vi "HeaderAction.vi"(0 "InstrClass":refnum<class "Spex.lvclass"> caption="DNL_LabVIEW Object in", 11 "error in (no error)":errorcluster caption="entrée d'erreur (pas d'erreur)") -> (4 "InstrClassOut":refnum<class "Spex.lvclass"> caption="DNL_LabVIEW Object out", 6 "DataNames":string[](array[string]), 8 "Instr Name":string, 10 "HeaderString":string, 14 "DisplayNames":string[](array[string]), 15 "error out":errorcluster caption="sortie d'erreur")   [LabVIEW 2019, in "Spex.lvclass"]
uses:
  Spex.lvclass
  C:/Programmes Labview/LabScanV1A/DevicesClass/BaseDevice/BaseDevice.lvclass
  Spex.lvclass/Spex.ctl
  BaseDevice/BaseDevice.lvclass
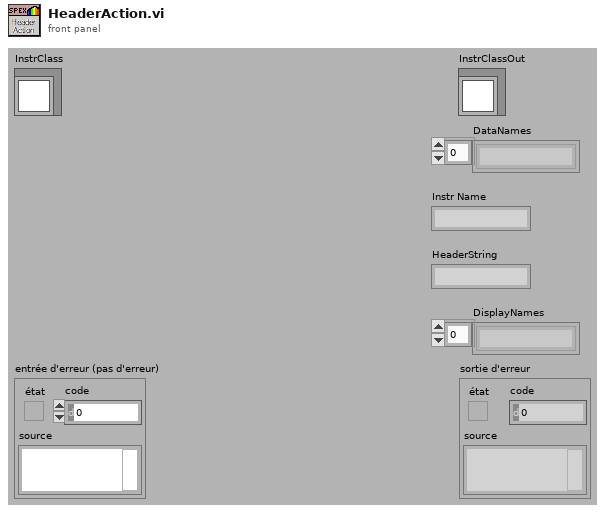
[diagram p1: front panel]
types:
  T1 = typedef "Spex.lvclass/Spex_Func.ctl" = enum16{"Position (nm)"}
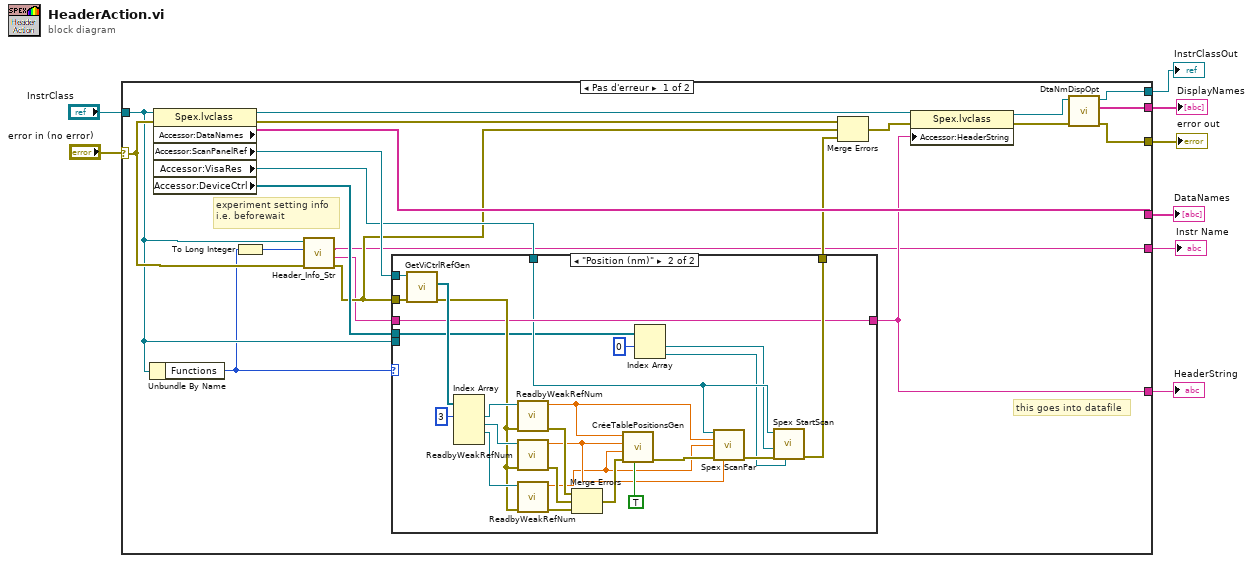
[diagram p0: block diagram]
diagram:
  n1 = case shown="Pas d'erreur" "error in (no error)" {
    selector: "error in (no error)" -> [w15 w57]
    tunnel: [w26 _] -> w7
    tunnel: [w29 _] -> w6
    tunnel: "InstrClass" -> [w14 w58]
    tunnel: [w24 w57] -> w4
    tunnel: [w23 w58] -> w2
    tunnel: [w10 _] -> w3
    tunnel: [w21 _] -> w1
    frame No Error {
      # "this goes into datafile"
      # "experiment setting info\ni.e. beforewait"
      n2 = Unbundle By Name(w14) -> ("Functions"=w13:T1)
      n3 = property class="Spex.lvclass"(reference=w14, error in=w15) -> (reference out=w28:refnum<class "Spex.lvclass">, error out=w27:errorcluster, "Accessor:DataNames"=w29:string[], "Accessor:ScanPanelRef"=w19:refnum<vi>, "Accessor:VisaRes"=w17:refnum<visa-resource-name>, "Accessor:DeviceCtrl"=w16:refnum<vi>[])
      n4 = To Long Integer(number=w13) -> (32bit integer=w12:i32)
      n5 = call-dynamic "Header_Info_Str.vi"("error in (no error)"=w15, "Functions"=w12, "DefaultDev in"=w14) -> ("error out"=w11:errorcluster, "HdrInfoStr"=w9:string, "InstrumentName"=w10:string)  [unwired: 5 in, 1 out]
      n6 = case shown="\"Position (nm)\"" w13 {
        tunnel: [w31 w38] -> w26
        tunnel: w9 -> [w31 w38]
        tunnel: w14 -> [_ _]
        tunnel: w19 -> [_ w52]
        tunnel: w11 -> [w30 w51]
        tunnel: [w30 w39] -> w18
        tunnel: w17 -> [_ w37]
        tunnel: w16 -> [_ w35]
        frame Default {
        }
        frame "Position (nm)" {
          n7 = call <userlib>:"GetViCtrlRefGen.vi"("ErrorIn(No Error)"=w51, "VIRef"=w52) -> ("sortie d'erreur"=w49:errorcluster, "ControlsRefs"=w50:refnum<vi>[])  [unwired: 7 in, 1 out]
          n8 = Index Array(array=w50, index #1=3 ("indice")) -> (element #1=w56:refnum<vi>, element #2=w55:refnum<vi>, element #3=w53:refnum<vi>)  [unwired: 3 in, 1 out]
          n9 = call <userlib>:"ReadbyWeakRefNum.vi"("error in"=w49, "Control Ref"=w56) -> ("error out"=w47:errorcluster, "Valeur"=w42:dbl)  [unwired: 8 in]
          n10 = call <userlib>:"ReadbyWeakRefNum.vi"("error in"=w49, "Control Ref"=w55) -> ("error out"=w45:errorcluster, "Valeur"=w41:dbl)  [unwired: 8 in]
          n11 = call <userlib>:"ReadbyWeakRefNum.vi"("error in"=w49, "Control Ref"=w53) -> ("error out"=w44:errorcluster, "Valeur"=w36:dbl)  [unwired: 8 in]
          n12 = Merge Errors(w47, w45, w44) -> (w46:errorcluster)
          n13 = call "CréeTablePositionsGen.vi"("InvInt"=TRUE, "error in (no error)"=w46, "Fin"=w36, "Increment"=w41, "Debut"=w42) -> ("error out"=w43:errorcluster)  [unwired: 4 in, 2 out]
          n14 = Index Array(array=w35, index #1=0 ("indice")) -> (element #1=w33:refnum<vi>, element #2=w32:refnum<vi>)  [unwired: 1 in]
          n15 = call <userlib>:"Spex ScanPar.vi"("Port"=w37, "Start(nm)"=w42, "End(nm)"=w36, "error in"=w43, "Step (nm)"=w41) -> ("error out"=w40:errorcluster)  [unwired: 10 in]
          n16 = call <userlib>:"Spex StartScan.vi"("Moving Ref"=w32, "error in"=w40, "Lambda Ref"=w33, "Port"=w37) -> ("error out"=w39:errorcluster)  [unwired: 5 in, 2 out]
        }
      }
      n17 = Merge Errors(w27, w11, w18) -> (w20:errorcluster)
      n18 = property class="Spex.lvclass"(reference=w28, error in=w20, "Accessor:HeaderString"=w26) -> (reference out=w22:refnum<class "Spex.lvclass">, error out=w25:errorcluster)
      n19 = call "DtaNmDispOpt.vi"("error in (no error)"=w25, "BaseDevice en entrée"=w22) -> ("error out"=w24:errorcluster, "DisplayNames"=w21:string[], "BaseDevice en sortie"=w23:refnum<class "Spex.lvclass">)  [unwired: 7 in]
    }
    frame Error {
    }
  }
  "error out" <- w4
  "InstrClassOut" <- w2
  "DataNames" <- w6
  "HeaderString" <- w7
  "Instr Name" <- w3
  "DisplayNames" <- w1
